vi "runtest Build DataFinder Query.vi"(7 "UserName":string, 8 "error in (no error)":errorcluster, 9 "Model Number":string, 10 "Serial Number":string) -> (0 "error out":errorcluster, 2 "Result TDM":path, 3 "Field Information":T1[](array[typedef]))   [LabVIEW 2011]
uses:
  server/DataFinder/eSearch Types.ctl
  server/DataFinder/DataFinder Comparisons.ctl
  server/DataFinder/Datafinder Query.ctl
  _cgi-lib/TDM_INDEX Record.ctl
  server/DD/lib/Query Queue.ctl
panel:
  out "Results":string[][](array[string])
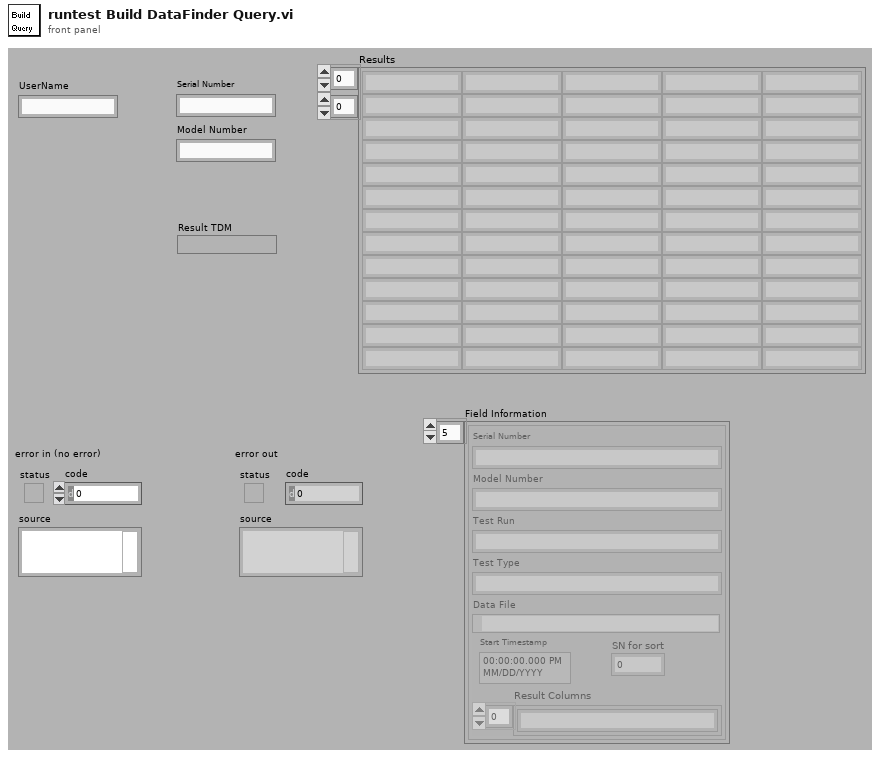
[diagram p1: front panel]
types:
  T1 = typedef "TDM_INDEX Record.ctl" = cluster{"Model Number":string, "SN for sort":i32, "Test Type":string, "Test Run":string, "Serial Number":string, "Start Timestamp":timestamp, "Data File":path, "Result Columns":string[]}
  T2 = typedef "Query Queue.ctl" = cluster{"UserName":string, "Search Parameters":T3[], "eSearch Type":T4, "Query Name (vbs)":string, "Response queue name":string, "Logic String":string}
  T3 = typedef "Datafinder Query.ctl" = cluster{"eSearch Types":T4, "Property Name":string, "DataFinder Comparisons":T5, "Property Value":string}
  T4 = typedef "eSearch Types.ctl" = enum16{"eSearchFile", "eSearchChannelGroup", "eSearchChannel"}
  T5 = typedef "DataFinder Comparisons.ctl" = enum16{"=", "<>", "<", "<=", ">", ">="}
  T6 = typedef "DIAdem Query Result.ctl" = cluster{"Results":string[][], "# of Items":i32, "Data Returned?":bool, "Result TDM":path, "Timed Out?":bool}
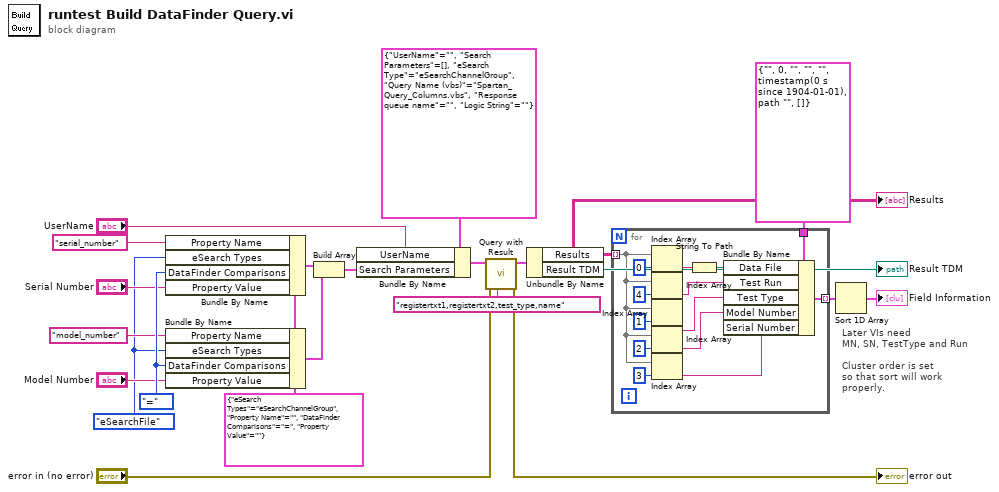
[diagram p0: block diagram]
diagram:
  w16 = DataFinder_Comparisons."=" ("DataFinder Comparisons")
  w2 = eSearch_Types."eSearchFile" ("eSearch Types")
  w10 = T3 {"eSearch Types"=enum."eSearchChannelGroup", "Property Name"="", "DataFinder Comparisons"=enum."=", "Property Value"=""} ("Data Finder Parameters")
  # "Later VIs need \nMN, SN, TestType and Run\n\nCluster order is set\nso that sort will work\nproperly."
  n1 = Bundle By Name(cluster=w10, "Property Name"="serial_number", "eSearch Types"=w2, "DataFinder Comparisons"=w16, "Property Value"="Serial Number") -> (w22:T3)
  n2 = Bundle By Name(cluster=w10, "Property Name"="model_number", "eSearch Types"=w2, "DataFinder Comparisons"=w16, "Property Value"="Model Number") -> (w13:T3)
  n3 = Build Array(w22, w13) -> (w4:T3[])
  n4 = Bundle By Name(cluster=T2 {"UserName"="", "Search Parameters"=[], "eSearch Type"=enum."eSearchChannelGroup", "Query Name (vbs)"="Spartan_Query_Columns.vbs", "Response queue name"="", "Logic String"=""} ("Query Parameter Data"), "UserName"="UserName", "Search Parameters"=w4) -> (w6:T2)
  n5 = call "Query with Result.vi"("result columns (comma list)"="registertxt1,registertxt2,test_type,name", "error in (no error)"="error in (no error)", "Query Parameter Data"=w6) -> ("error out"=→"error out":errorcluster, "Query Return Data"=w9:T6)  [unwired: 1 in, 6 out]
  n6 = Unbundle By Name(w9) -> ("Results"=w1:string[][], "Result TDM"=→"Result TDM":path)
  "Results" <- w1
  n7 = for {
    tunnel: w1 -> [w24] mode=indexing
    tunnel: T1 {"Model Number"="", "SN for sort"=0, "Test Type"="", "Test Run"="", "Serial Number"="", "Start Timestamp"=timestamp(0 s since 1904-01-01), "Data File"=path "", "Result Columns"=[]} ("Station Information") -> [w36]
    tunnel: [w31] -> w19 mode=indexing
    n8 = Index Array(array=w24, index=0) -> (element=w33:string)
    n9 = Index Array(array=w24, index=4) -> (element=w32:string)
    n10 = Index Array(array=w24, index=1) -> (element=w23:string)
    n11 = Index Array(array=w24, index=2) -> (element=w28:string)
    n12 = Index Array(array=w24, index=3) -> (element=w27:string)
    n13 = String To Path(string=w33) -> (path=w26:path)
    n14 = Bundle By Name(cluster=w36, "Data File"=w26, "Test Run"=w32, "Test Type"=w23, "Model Number"=w28, "Serial Number"=w27) -> (w31:T1)
  }
  n15 = Sort 1D Array(array=w19) -> (sorted array=→"Field Information":T1[])
